vi "getFrameSize.vi"(8 "error in":T1, 11 "channel":i32) -> (0 "error out":T1, 3 "FrameSize":i32)   [LabVIEW 2016]
doc: "\"FrameSize\" is an integer, which tells you how many data points will be retrieved from a given data channel (input). This information is usually required by getData.vi. Please use this VI to calculate the frame size of a channel instead of doing it manually."
uses:
  Controls/Error_Out.ctl
  Files_ASC500/DLL/daisybase.dll
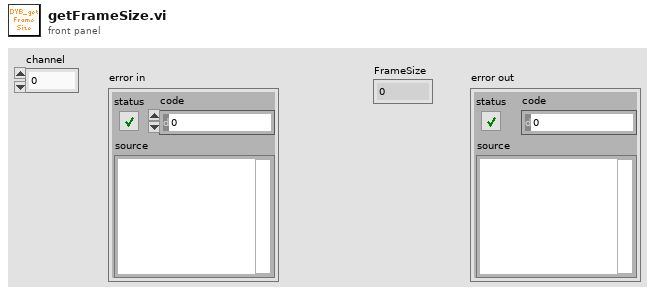
[diagram p1: front panel]
types:
  T1 = typedef "Error_Out.ctl" = errorcluster
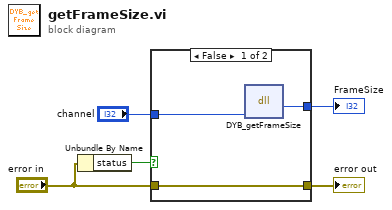
[diagram p0: block diagram]
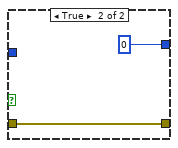
[diagram p2: hidden frame]
diagram:
  n1 = Unbundle By Name("error in") -> ("status"=w5:bool)
  n2 = case shown="False" w5 {
    tunnel: "channel" -> [w8 _]
    tunnel: "error in" -> [w7 w10]
    tunnel: [w7 w10] -> w2
    tunnel: [w6 0 ("FrameSize")] -> w1
    frame False {
      n3 = dll-call lib="G:/SCMOperations/Share/ELE/Produkt Information/ASC500/04 Remote Control/02 development versions/2018Nov06/Files_ASC500/DLL/daisybase.dll" fn="DYB_getFrameSize"("channel"=w8) -> ("FrameSize"=w6:i32)  [unwired: 4 in, 2 out]
    }
    frame True {
    }
  }
  "error out" <- w2
  "FrameSize" <- w1
